vi "Apply_Filters_to_Tracks-3.vi"(8 "error IN":errorcluster, 10 "[IN] Control Parameters":T4, 11 "[IN] Movie Values":T3 {"Particle Fil Setups"."Type of particle filter"."Measurement Parameter" items=["Center of Mass X", "Center of Mass Y", "First Pixel X", "First Pixel Y", "Bounding Rect Left", "Bounding Rect Top", "Bounding Rect Right", "Bounding Rect Bottom", "Max Feret Diameter Start X", "Max Feret Diameter Start Y", "Max Feret Diameter End X", "Max Feret Diameter End Y", "Max Horiz. Segment Length Left", "Max Horiz. Segment Length Right", "Max Horiz. Segment Length Row", "-", "Bounding Rect Width", "Bounding Rect Height", "Bounding Rect Diagonal", "Perimeter", "Convex Hull Perimeter", "Holes' Perimeter", "Max Feret Diameter", "Equivalent Ellipse Major Axis", "Equivalent Ellipse Minor Axis", "Equivalent Ellipse Minor Axis (Feret)", "Equivalent Rect Long Side", "Equivalent Rect Short Side", "Equivalent Rect Diagonal", "Equivalent Rect Short Side (Feret)", "Average Horiz. Segment Length", "Average Vert. Segment Length", "Hydraulic Radius", "Waddel Disk Diameter", "-", "Area", "Holes' Area", "Particle & Holes' Area", "Convex Hull Area", "Image Area", "-", "Number of Holes", "Number of Horiz. Segments", "Number of Vert. Segments", "-", "Orientation", "Max Feret Diameter Orientation", "-", "% Area/Image Area", "% Area/(Particle & Holes' Area)", "Ratio of Equivalent Ellipse Axes", "Ratio of Equivalent Rect Sides", "-", "Elongation Factor", "Compactness Factor", "Heywood Circularity Factor", "Type Factor", "-", "Sum X", "Sum Y", "Sum XX", "Sum XY", "Sum YY", "Sum XXX", "Sum XXY", "Sum XYY", "Sum YYY", "-", "Moment of Inertia XX", "Moment of Inertia XY", "Moment of Inertia YY", "Moment of Inertia XXX", "Moment of Inertia XXY", "Moment of Inertia XYY", "Moment of Inertia YYY", "Norm. Moment of Inertia XX", "Norm. Moment of Inertia XY", "Norm. Moment of Inertia YY", "Norm. Moment of Inertia XXX", "Norm. Moment of Inertia XXY", "Norm. Moment of Inertia XYY", "Norm. Moment of Inertia YYY", "Hu Moment 1", "Hu Moment 2", "Hu Moment 3", "Hu Moment 4", "Hu Moment 5", "Hu Moment 6", "Hu Moment 7"]}) -> (0 "error OUT":errorcluster, 1 "[OUT] Filtered Tracks":T1(array[cluster]), 2 "[OUT] # Displ \nafter Filtration":i32, 3 "[OUT] Filtered Movie Values":T3 {"Particle Fil Setups"."Type of particle filter"."Measurement Parameter" items=["Center of Mass X", "Center of Mass Y", "First Pixel X", "First Pixel Y", "Bounding Rect Left", "Bounding Rect Top", "Bounding Rect Right", "Bounding Rect Bottom", "Max Feret Diameter Start X", "Max Feret Diameter Start Y", "Max Feret Diameter End X", "Max Feret Diameter End Y", "Max Horiz. Segment Length Left", "Max Horiz. Segment Length Right", "Max Horiz. Segment Length Row", "-", "Bounding Rect Width", "Bounding Rect Height", "Bounding Rect Diagonal", "Perimeter", "Convex Hull Perimeter", "Holes' Perimeter", "Max Feret Diameter", "Equivalent Ellipse Major Axis", "Equivalent Ellipse Minor Axis", "Equivalent Ellipse Minor Axis (Feret)", "Equivalent Rect Long Side", "Equivalent Rect Short Side", "Equivalent Rect Diagonal", "Equivalent Rect Short Side (Feret)", "Average Horiz. Segment Length", "Average Vert. Segment Length", "Hydraulic Radius", "Waddel Disk Diameter", "-", "Area", "Holes' Area", "Particle & Holes' Area", "Convex Hull Area", "Image Area", "-", "Number of Holes", "Number of Horiz. Segments", "Number of Vert. Segments", "-", "Orientation", "Max Feret Diameter Orientation", "-", "% Area/Image Area", "% Area/(Particle & Holes' Area)", "Ratio of Equivalent Ellipse Axes", "Ratio of Equivalent Rect Sides", "-", "Elongation Factor", "Compactness Factor", "Heywood Circularity Factor", "Type Factor", "-", "Sum X", "Sum Y", "Sum XX", "Sum XY", "Sum YY", "Sum XXX", "Sum XXY", "Sum XYY", "Sum YYY", "-", "Moment of Inertia XX", "Moment of Inertia XY", "Moment of Inertia YY", "Moment of Inertia XXX", "Moment of Inertia XXY", "Moment of Inertia XYY", "Moment of Inertia YYY", "Norm. Moment of Inertia XX", "Norm. Moment of Inertia XY", "Norm. Moment of Inertia YY", "Norm. Moment of Inertia XXX", "Norm. Moment of Inertia XXY", "Norm. Moment of Inertia XYY", "Norm. Moment of Inertia YYY", "Hu Moment 1", "Hu Moment 2", "Hu Moment 3", "Hu Moment 4", "Hu Moment 5", "Hu Moment 6", "Hu Moment 7"]}, 4 "[OUT] Filtered Tracks\nw/t Problems":T1(array[cluster]))   [LabVIEW 2017]
doc: "This \"high-level\" subVI encloses all filters which operate on the found tracks for selecting linear (processive) and sufficiently long tracks"
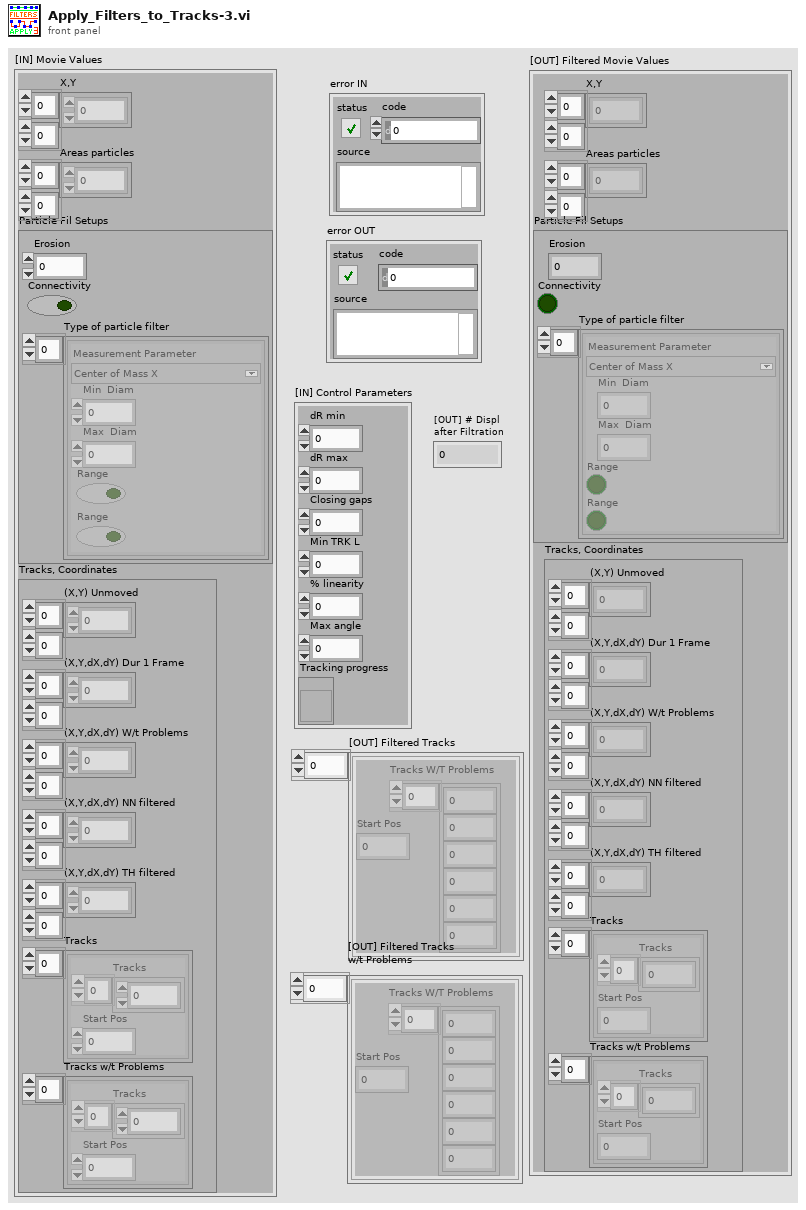
[diagram p1: front panel]
types:
  T1 = cluster{"Tracks W/T Problems":dbl[], "Start Pos":i32}[]
  T2 = typedef "Particle Parameters" = i32
  T3 = cluster{"X,Y":dbl[][], "Areas particles":dbl[][], "Particle Fil Setups":cluster{"Erosion":i32, "Connectivity ":bool, "Type of particle filter":cluster{"Measurement Parameter":T2, "Min  Diam":dbl, "Max  Diam":dbl, "Range":bool, "Range":bool}[]}, "Tracks, Coordinates":cluster{"(X,Y) Unmoved":dbl[][], "(X,Y,dX,dY) Dur 1 Frame":dbl[][], "(X,Y,dX,dY) W/t Problems":dbl[][], "(X,Y,dX,dY) NN filtered":dbl[][], "(X,Y,dX,dY) TH filtered":dbl[][], "Tracks":cluster{"Tracks":dbl[], "Start Pos":i32}[], "Tracks w/t Problems":cluster{"Tracks":dbl[], "Start Pos":i32}[]}}
  T4 = cluster{"dR min ":dbl, "dR max ":dbl, "Closing gaps":i32, "Min TRK L":i32, "% linearity":i32, "Max angle":dbl, "Tracking progress":refnum<vi>}
  T5 = cluster{"X,Y":dbl[][], "Areas particles":dbl[][], "Particle Fil Setups":cluster{"Erosion":i32, "Connectivity ":bool, "Type of particle filter":cluster{"Measurement Parameter":T2, "Min  Diam":dbl, "Max  Diam":dbl, "Range":bool, "Range":bool}[]}, "Tracks, Coordinates":cluster{"(X,Y) Unmoved":dbl[][], "(X,Y,dX,dY) Dur 1 Frame":dbl[][], "(X,Y,dX,dY) whole (dt>1)":dbl[][], "(X,Y,dX,dY) NN filtered":dbl[][], "(X,Y,dX,dY) TH filtered":dbl[][], "Tracks + Starting Position":cluster{"Tracks":dbl[], "Start Pos":i32}[]}}
  T6 = cluster{"(X,Y) Unmoved":dbl[][], "(X,Y,dX,dY) Dur 1 Frame":dbl[][], "(X,Y,dX,dY) W/t Problems":dbl[][], "(X,Y,dX,dY) NN filtered":dbl[][], "(X,Y,dX,dY) TH filtered":dbl[][], "Tracks":cluster{"Tracks":dbl[], "Start Pos":i32}[], "Tracks w/t Problems":cluster{"Tracks":dbl[], "Start Pos":i32}[]}
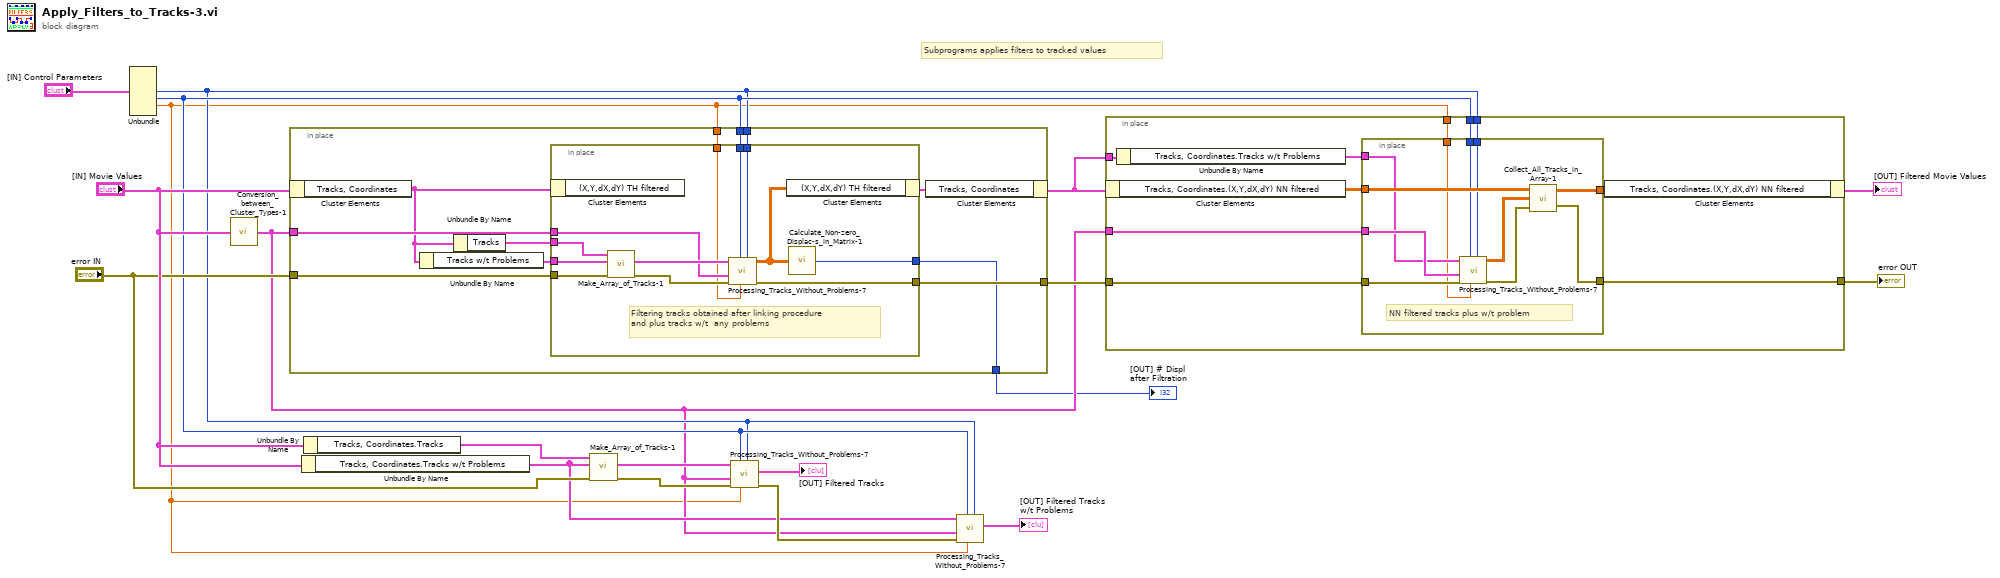
[diagram p0: block diagram]
diagram:
  # "Subprograms applies filters to tracked values"
  n1 = Unbundle("[IN] Control Parameters") -> ("Min TRK L"=w5:i32, "% linearity"=w6:i32, "Max angle"=w3:dbl)  [unwired: 4 out]
  n2 = call "Conversion_between_Cluster_Types-1.vi"("[IN] New Movie Values"="[IN] Movie Values") -> ("[OUT] Old Movie Values"=w4:T5)
  n3 = in-place {
    in-place-border: "error IN" -> [w30]
    in-place-border: w4 -> [w29]
    in-place-border: w6 -> [w28]
    in-place-border: w5 -> [w27]
    in-place-border: w3 -> [w26]
    in-place-border: [w24] -> w18
    in-place-border: [w20] -> w1
    n4 = in-place-cluster #1("[IN] Movie Values") -> ("Tracks, Coordinates"=w22:T6)
    n5 = Unbundle By Name(w22) -> ("Tracks w/t Problems"=w21:cluster{"Tracks":dbl[], "Start Pos":i32}[])
    n6 = Unbundle By Name(w22) -> ("Tracks"=w23:cluster{"Tracks":dbl[], "Start Pos":i32}[])
    n7 = in-place {
      in-place-border: w30 -> [w42]
      in-place-border: w29 -> [w36]
      in-place-border: w28 -> [w39]
      in-place-border: w27 -> [w38]
      in-place-border: w26 -> [w32]
      in-place-border: [w34] -> w24
      in-place-border: w23 -> [w41]
      in-place-border: w21 -> [w40]
      in-place-border: [w31] -> w20
      # "Filtering tracks obtained after linking procedure \nand plus tracks w/t  any problems"
      n8 = in-place-cluster #2(w22) -> ()  [unwired: 1 out]
      n9 = call "Make_Array_of_Tracks-1.vi"("error IN"=w42, "[IN] Filtered Tracks w/t Problems"=w40, "[IN] Filtered Tracks with Problems"=w41) -> ("error OUT"=w35:errorcluster, "[OUT] Array of tracks"=w37:cluster{"Tracks":dbl[], "Start Pos":i32}[])  [unwired: 3 in]
      n10 = call "Processing_Tracks_Without_Problems-7.vi"("[IN] Min TRK L"=w38, "[IN] Max angle between \ntwo displacements"=w32, "[IN] % linearity"=w39, "error IN"=w35, "[IN] Movie Values"=w36, "[IN] Tracks w/t Problems"=w37) -> ("error OUT"=w34:errorcluster, "[OUT] Frame-to-Frame Displacements\n Extract From Tracks"=w33:dbl[][])  [unwired: 3 in, 1 out]
      n11 = in-place-cluster #2("(X,Y,dX,dY) TH filtered"=w33) -> (w25:T6)
      n12 = call "Calculate_Non-zero_Displac-s_in_Matrix-1.vi"("[IN] Displacements \nFrm-to-Frm In Cols"=w33) -> ("[OUT] Number of \n(X,Y,dX,dY) displ-s"=w31:i32)
    }
    n13 = in-place-cluster #1("Tracks, Coordinates"=w25) -> (w15:T3)
  }
  "[OUT] # Displ \nafter Filtration" <- w1
  n14 = Unbundle By Name("[IN] Movie Values") -> ("Tracks, Coordinates.Tracks w/t Problems"=w7:cluster{"Tracks":dbl[], "Start Pos":i32}[])
  n15 = Unbundle By Name("[IN] Movie Values") -> ("Tracks, Coordinates.Tracks"=w13:cluster{"Tracks":dbl[], "Start Pos":i32}[])
  n16 = call "Make_Array_of_Tracks-1.vi"("error IN"="error IN", "[IN] Filtered Tracks w/t Problems"=w7, "[IN] Filtered Tracks with Problems"=w13) -> ("error OUT"=w10:errorcluster, "[OUT] Array of tracks"=w11:cluster{"Tracks":dbl[], "Start Pos":i32}[])  [unwired: 3 in]
  n17 = call "Processing_Tracks_Without_Problems-7.vi"("[IN] Min TRK L"=w5, "[IN] Max angle between \ntwo displacements"=w3, "[IN] % linearity"=w6, "error IN"=w10, "[IN] Movie Values"=w4, "[IN] Tracks w/t Problems"=w11) -> ("error OUT"=w8:errorcluster, "[OUT] Filtered Tracks"=→"[OUT] Filtered Tracks":T1)  [unwired: 3 in, 1 out]
  n18 = call "Processing_Tracks_Without_Problems-7.vi"("[IN] Min TRK L"=w5, "[IN] Max angle between \ntwo displacements"=w3, "[IN] % linearity"=w6, "error IN"=w8, "[IN] Movie Values"=w4, "[IN] Tracks w/t Problems"=w7) -> ("[OUT] Filtered Tracks"=→"[OUT] Filtered Tracks\nw/t Problems":T1)  [unwired: 3 in, 2 out]
  n19 = in-place {
    in-place-border: w18 -> [w52]
    in-place-border: w4 -> [w51]
    in-place-border: w6 -> [w50]
    in-place-border: w5 -> [w49]
    in-place-border: w3 -> [w48]
    in-place-border: [w47] -> w17
    in-place-border: w15 -> [w44]
    n20 = in-place-cluster #3(w15) -> ("Tracks, Coordinates.(X,Y,dX,dY) NN filtered"=w46:dbl[][])
    n21 = Unbundle By Name(w44) -> ("Tracks, Coordinates.Tracks w/t Problems"=w43:cluster{"Tracks":dbl[], "Start Pos":i32}[])
    n22 = in-place {
      in-place-border: w52 -> [w57]
      in-place-border: w51 -> [w56]
      in-place-border: w50 -> [w60]
      in-place-border: w49 -> [w59]
      in-place-border: w48 -> [w54]
      in-place-border: [w61] -> w47
      in-place-border: w46 -> [w63]
      in-place-border: [w62] -> w45
      in-place-border: w43 -> [w55]
      # "NN filtered tracks plus w/t problem"
      n23 = call "Processing_Tracks_Without_Problems-7.vi"("[IN] Min TRK L"=w59, "[IN] Max angle between \ntwo displacements"=w54, "[IN] % linearity"=w60, "error IN"=w57, "[IN] Movie Values"=w56, "[IN] Tracks w/t Problems"=w55) -> ("error OUT"=w58:errorcluster, "[OUT] Frame-to-Frame Displacements\n Extract From Tracks"=w53:dbl[][])  [unwired: 3 in, 1 out]
      n24 = call "Collect_All_Tracks_in_Array-1.vi"("error in"=w58, "Tracks(Frames) #2"=w53, "Tracks(Frames) #1"=w63) -> ("error out"=w61:errorcluster, "[OUT] Collected Tracks"=w62:dbl[][])
    }
    n25 = in-place-cluster #3("Tracks, Coordinates.(X,Y,dX,dY) NN filtered"=w45) -> (→"[OUT] Filtered Movie Values":T3)
  }
  "error OUT" <- w17
